vi "Explode.vi"(11 "String In":string) -> (2 "Exploded?":bool, 3 "String Out":string)   [LabVIEW 2021]
uses:
  <vilib>/regexp/Match Regular Expression.xnode
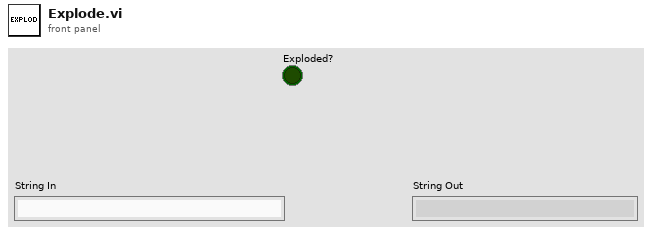
[diagram p1: front panel]
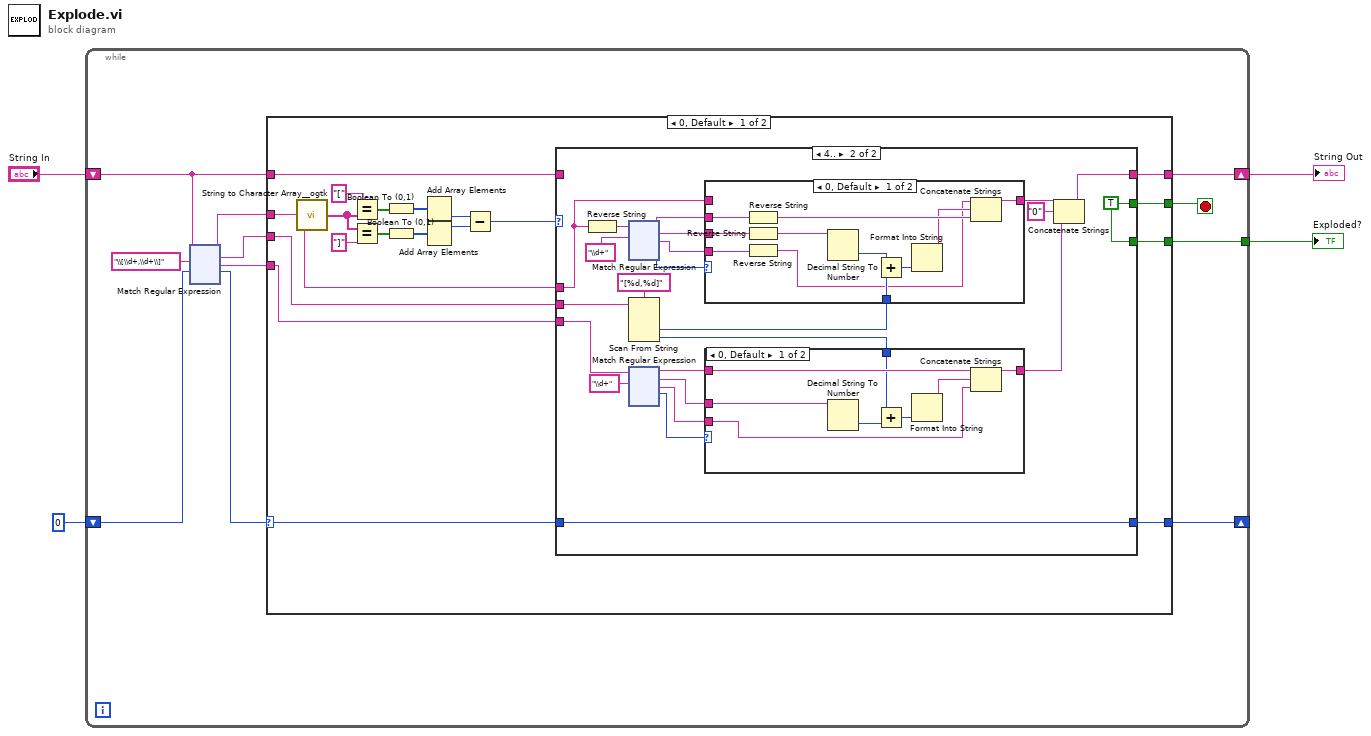
[diagram p0: block diagram]
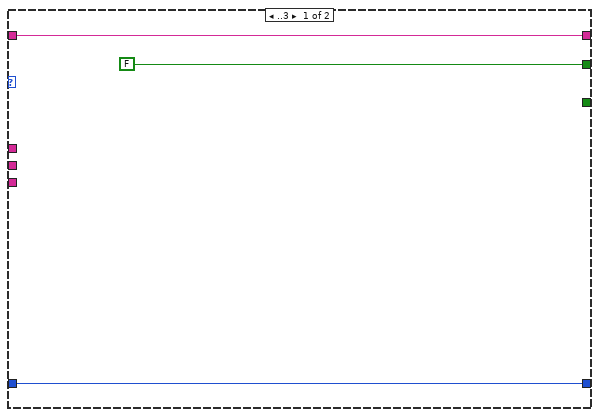
[diagram p2: hidden frame]
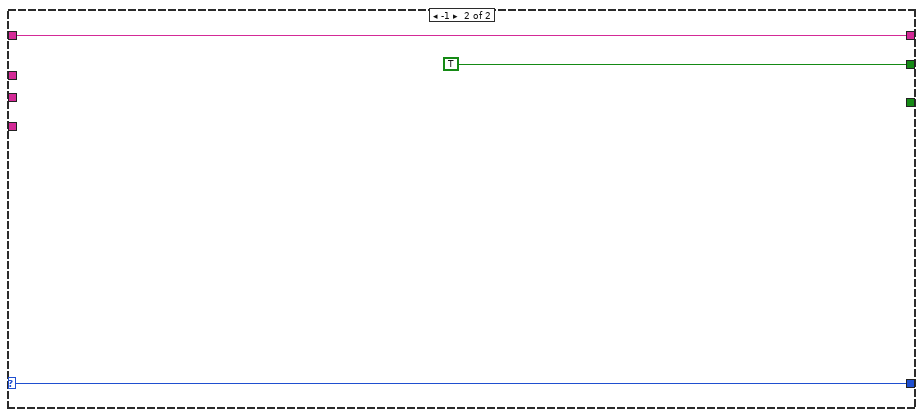
[diagram p5: hidden frame]
diagram:
  n1 = while {
    shift-right: [w13] -> w3
    shift-left: "String In" -> [w14]
    shift-right: [w7] -> _
    shift-left: 0 -> [w8]
    tunnel: [w5] -> w1
    stop <- w9 stop-if-true
    n2 = xnode "Match Regular Expression"("input string"=w14, "regular expression"="\\[\\d+,\\d+\\]", "offset (0)"=w8) -> ("before match"=w11:string, "whole match"=w10:string, "after match"=w12:string, "offset past match"=w6:i32)  [unwired: 3 in, 1 out]
    n3 = case shown="0, Default" w6 {
      selector: w6 -> [w22 w316]
      tunnel: w14 -> [w25 w318]
      tunnel: [w24 w318] -> w13
      tunnel: w12 -> [w16 _]
      tunnel: w11 -> [w18 _]
      tunnel: w10 -> [w17 _]
      tunnel: [w23 TRUE] -> w9
      tunnel: [w21 w316] -> w7
      tunnel: [w20 _] -> w5
      frame 0, Default {
        n4 = call <userlib>:"String to Character Array__ogtk.vi"("Input String"=w18) -> ("Character Array"=w33:string[])
        n5 = Equal?(x="[", y=w33) -> (x = y?=w31:bool[])
        n6 = Equal?(x=w33, y="]") -> (x = y?=w26:bool[])
        n7 = Boolean To (0,1)(Boolean=w31) -> (0, 1=w29:i16[])
        n8 = Boolean To (0,1)(Boolean=w26) -> (0, 1=w28:i16[])
        n9 = Add Array Elements(numeric array=w29) -> (sum=w30:i16)
        n10 = Add Array Elements(numeric array=w28) -> (sum=w27:i16)
        n11 = Subtract(x=w30, y=w27) -> (x-y=w19:i16)
        n12 = case shown="4.." w19 {
          tunnel: w25 -> [w37 _]
          tunnel: [w37 w44] -> w24
          tunnel: [FALSE w59] -> w23
          tunnel: w22 -> [w35 w60]
          tunnel: [w35 w60] -> w21
          tunnel: [_ w59] -> w20
          tunnel: w18 -> [_ w48]
          tunnel: w17 -> [_ w57]
          tunnel: w16 -> [_ w56]
          frame ..3 {
          }
          frame 4.. {
            w59 = TRUE
            n13 = Reverse String(1:w48) -> (0:w53:string)
            n14 = xnode "Match Regular Expression"("input string"=w53, "regular expression"="\\d+") -> ("before match"=w51:string, "whole match"=w52:string, "after match"=w50:string, "offset past match"=w49:i32)  [unwired: 4 in, 1 out]
            n15 = Scan From String(format string="[%d,%d]" ("regular expression"), input string=w57) -> (output 1=w47:i32, output 2=w39:i32)  [unwired: 4 in, 3 out]
            n16 = xnode "Match Regular Expression"("input string"=w56, "regular expression"="\\d+") -> ("before match"=w41:string, "whole match"=w40:string, "after match"=w43:string, "offset past match"=w42:i32)  [unwired: 4 in, 1 out]
            n17 = case shown="0, Default" w49 {
              tunnel: w52 -> [w80 _]
              tunnel: w51 -> [w79 _]
              tunnel: w50 -> [w78 _]
              tunnel: w48 -> [_ w81]
              tunnel: [w70 w81] -> w46
              tunnel: w47 -> [w76 _]
              frame 0, Default {
                n18 = Reverse String(1:w79) -> (0:w73:string)
                n19 = Reverse String(1:w80) -> (0:w77:string)
                n20 = Reverse String(1:w78) -> (0:w71:string)
                n21 = Decimal String To Number(string=w77) -> (number=w75:i32)  [unwired: 2 in, 1 out]
                n22 = Add(x=w75, y=w76) -> (x+y=w74:i32)
                n23 = Format Into String(w74) -> (resulting string=w72:string)  [unwired: 3 in, 1 out]
                n24 = Concatenate Strings(w71, w72, w73) -> (w70:string)
              }
              frame -1 {
              }
            }
            n25 = case shown="0, Default" w42 {
              tunnel: w40 -> [w68 _]
              tunnel: w43 -> [w61 _]
              tunnel: w41 -> [w63 w69]
              tunnel: [w64 w69] -> w38
              tunnel: w39 -> [w62 _]
              frame 0, Default {
                n26 = Decimal String To Number(string=w68) -> (number=w67:i32)  [unwired: 2 in, 1 out]
                n27 = Add(x=w62, y=w67) -> (x+y=w66:i32)
                n28 = Format Into String(w66) -> (resulting string=w65:string)  [unwired: 3 in, 1 out]
                n29 = Concatenate Strings(w63, w65, w61) -> (w64:string)
              }
              frame -1 {
              }
            }
            n30 = Concatenate Strings(w46, "0" ("string"), w38) -> (w44:string)
          }
        }
      }
      frame -1 {
      }
    }
  }
  "String Out" <- w3
  "Exploded?" <- w1
